vi "Do.vi"(8 "error in (no error)":errorcluster, 10 "Actor in":refnum<class "Actor.lvclass">, 11 "ControlMouseEnterMsg":refnum<class "ControlMouseEnterMsg.lvclass">) -> (0 "error out":errorcluster, 2 "Actor out":refnum<class "Actor.lvclass">)   [LabVIEW 2015, in "ActorEvents.lvlib" / "ControlMouseEnterMsg.lvclass"]
doc: "(<B>Filename</B>: Actor Framework.lvlib:Message.lvclass:Do.vi)\n\nDefines what a message does when it is received by an actor. Generally, a message instructs an actor to invoke one of its methods. By default, this method does nothing. A child class must override it to define behavior. Create a child class by using the Actor Framework Message Maker dialog box.\n\n<License>\nCopyright © 2017 Composed Systems, LLC | All rights reserved\nwww.composed.io\n\nAuthor: Ethan Stern <ethan.stern@composed.io>\n\nThis software is provided \"AS IS\" WITHOUT WARRANTIES, either express or implied, AND IS FOR EDUCATIONAL PURPOSES ONLY.\n</License>"
uses:
  ControlMouseEnterMsg.lvclass
  <vilib>/ActorFramework/Actor/Actor.lvclass
  IEventAggregator/IEventAggregator.lvclass
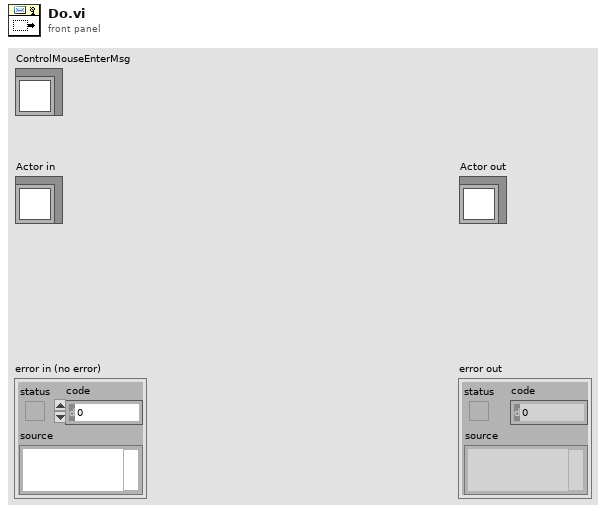
[diagram p1: front panel]
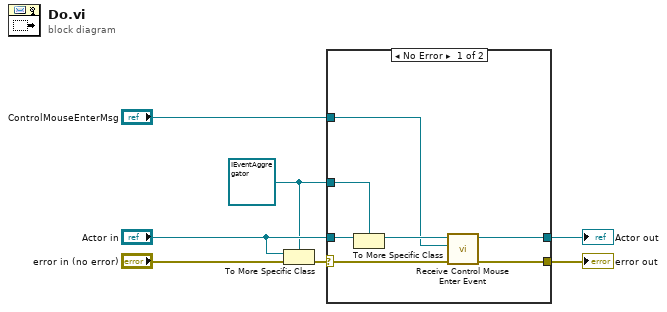
[diagram p0: block diagram]
diagram:
  w1 = refnum<class "IEventAggregator.lvclass"> refnum ("Actor in")
  n1 = To More Specific Class(target class=w1, reference="Actor in", error in="error in (no error)") -> (error out=w7:errorcluster)  [unwired: 1 out]
  n2 = case shown="No Error" w7 {
    selector: w7 -> [w10 w16]
    tunnel: [w9 w16] -> w6
    tunnel: [w11 w15] -> w5
    tunnel: "Actor in" -> [w14 w15]
    tunnel: w1 -> [w13 _]
    tunnel: "ControlMouseEnterMsg" -> [w8 _]
    frame No Error {
      n3 = To More Specific Class(target class=w13, reference=w14) -> (specific class reference=w12:refnum<class "IEventAggregator.lvclass">)  [unwired: 1 in, 1 out]
      n4 = call-dynamic "Receive Control Mouse Enter Event.vi"("error in (no error)"=w10, "ControlMouseEnterMsg"=w8, "IEventAggregator In"=w12) -> ("error out"=w9:errorcluster, "IEventAggregator Out"=w11:refnum<class "IEventAggregator.lvclass">)  [unwired: 7 in]
    }
    frame Error {
      # "If type check fails, pass the\noriginal object out again."
    }
  }
  "error out" <- w6
  "Actor out" <- w5
